vi "Magic Transparent Color Constant.vi"() -> (3 "Magic transparent color constant":u32(colorbox)=16777214)   [LabVIEW 2021, in "lv_icon.lvlib"]
doc: "This is the magic transparent color constant of the Icon Editor."
uses:
  lv_icon.lvlib
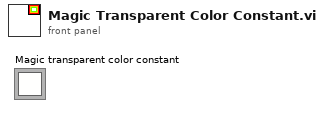
[diagram p1: front panel]
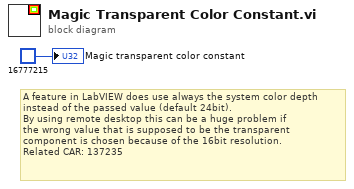
[diagram p0: block diagram]
diagram:
  # "A feature in LabVIEW does use always the system color depth\ninstead of the passed value (default 24bit).\nBy using remote desktop this can be a huge problem if\nthe wrong value that is supposed to be the transparent\ncomponent is chosen because of the 16bit resolution.\nRelated CAR: 137235"
  "Magic transparent color constant" <- u32 16777215 ("Color")
